vi "Load Configuration File.vi"() -> ()   [LabVIEW 2012]
panel:
  out "text":string
  out "Write OK":bool
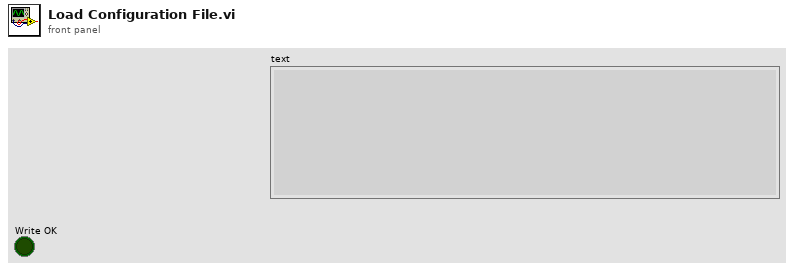
[diagram p1: front panel]
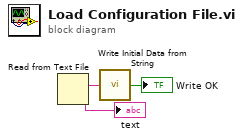
[diagram p0: block diagram]
diagram:
  n1 = Read from Text File() -> (text=w1:string)  [unwired: 4 in, 3 out]
  "text" <- w1
  n2 = call "Write Initial Data from String.vi"("Data"=w1) -> ("Write OK"=→"Write OK":bool)
